vi "hong_wai_ce_ju-5.12.vi"() -> ()   [LabVIEW 2015]
uses:
  <vilib>/DAQmx/read.llb/DAQmx Read (Analog DBL 1Chan 1Samp).vi
  <vilib>/DAQmx/create/channels.llb/DAQmx Create Channel (AI-Voltage-Basic).vi
  <vilib>/DAQmx/miscellaneous.llb/DAQmx Fill In Error Info.vi
  <vilib>/ptbypt/NI_PtbyPt.lvlib
panel:
  out "Numeric":dbl
  out "距离":dbl(knob) scale=0.0..150.0
  out "error out":errorcluster
  in  "Channels":tag
  in  "stop":bool
  # "红外测距"
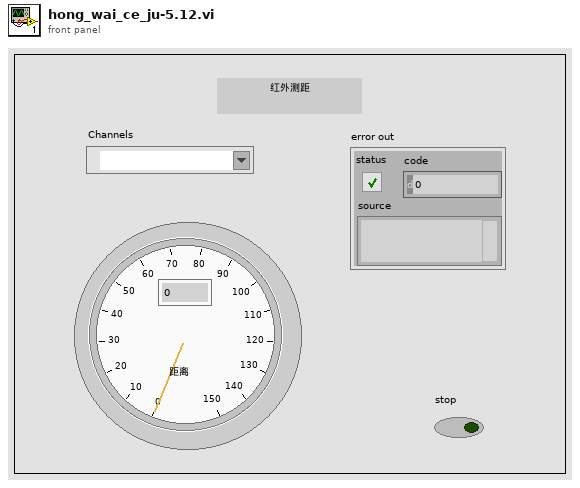
[diagram p1: front panel]
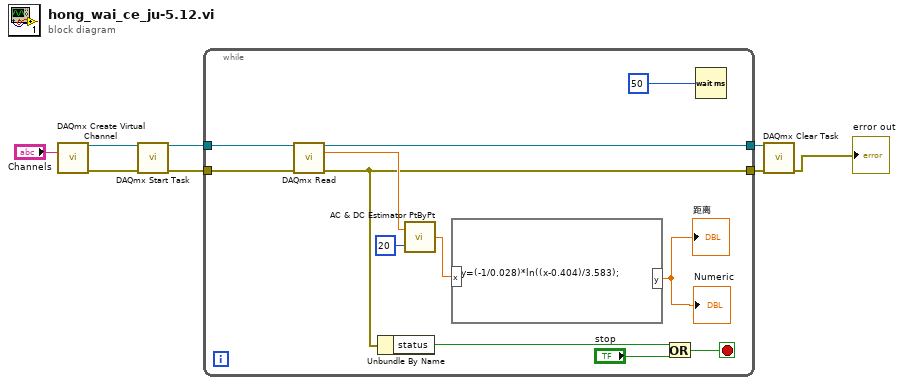
[diagram p0: block diagram]
diagram:
  n1 = call-poly <vilib>:"DAQmx Create Virtual Channel.vi"("physical channels"="Channels") -> ("task out"=w6:refnum<k21>, "error out"=w4:errorcluster)  [unwired: 13 in]
  n2 = call <vilib>:"DAQmx Start Task.vi"("task/channels in"=w6, "error in"=w4) -> ("task out"=w5:refnum<k21>, "error out"=w3:errorcluster)  [unwired: 12 in]
  n3 = while {
    tunnel: [w19] -> w8
    tunnel: [w14] -> w7
    tunnel: w5 -> [w18]
    tunnel: w3 -> [w17]
    stop <- w13 stop-if-true
    n4 = call-poly <vilib>:"DAQmx Read.vi"("task/channels in"=w18, "error in"=w17) -> ("task out"=w19:refnum<k21>, "data"=w16:dbl, "error out"=w14:errorcluster)  [unwired: 11 in]
    n5 = Unbundle By Name(w14) -> ("status"=w12:bool)
    n6 = call <vilib>:"AC & DC Estimator PtByPt.vi"("signal"=w16, "sample length"=20) -> ("DC estimate (V)"=w10:dbl)  [unwired: 1 in, 2 out]
    n7 = formula code="y=(-1/0.028)*ln((x-0.404)/3.583);"("x"=w10) -> ("y"=→"距离" →"Numeric":dbl)
    n8 = Or(x=w12, y="stop") -> (x .or. y?=w13:bool)
    n9 = Wait (ms)(milliseconds to wait=u32 50) -> ()  [unwired: 1 out]
  }
  n10 = call <vilib>:"DAQmx Clear Task.vi"("task in"=w8, "error in"=w7) -> ("error out"=→"error out":errorcluster)  [unwired: 13 in]
